vi "Team Colors.vi"() -> (2 "Team Colors":u32[](array[colorbox])=[6618880, 16711680, 255, 16776960, 16711935, 65535, 16744448, 8421631, 16711808, 16448250])   [LabVIEW 2020, in "SquareBattle.lvlib"]
uses:
  SquareBattle.lvlib
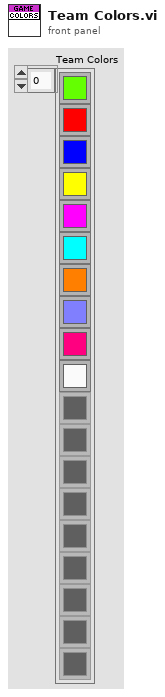
[diagram p1: front panel]
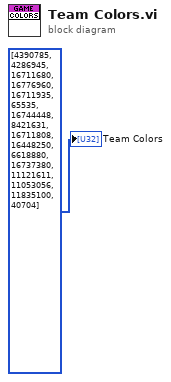
[diagram p0: block diagram]
diagram:
  "Team Colors" <- u32[] [4390785, 4286945, 16711680, 16776960, 16711935, 65535, 16744448, 8421631, 16711808, 16448250, 6618880, 16737380, 11121611, 11053056, 11835100, 40704]
